vi "Q1.vi"() -> ()   [LabVIEW 2018]
uses:
  <vilib>/Analysis/geometry.llb/Point in Polygon Position.ctl
  <vilib>/Analysis/geometry.llb/Point in Polygon (Array).vi
  <vilib>/Analysis/NI_AAL_Geometry.lvlib
panel:
  out "Pendiente":dbl[](array[numeric])
  out "Puntoy":dbl[](array[numeric])
  out "Puntox":dbl[](array[numeric])
  out "Position":T1[](array[typedef]) items=["Inside", "On Boundary", "Outside"]
  out "Limite del poligono superado":bool[](array[boolean])
  out "XY Graph":cluster{"Puntox":dbl[], "Puntoy":dbl[]}[](graph)
  in  "Cluster":T2
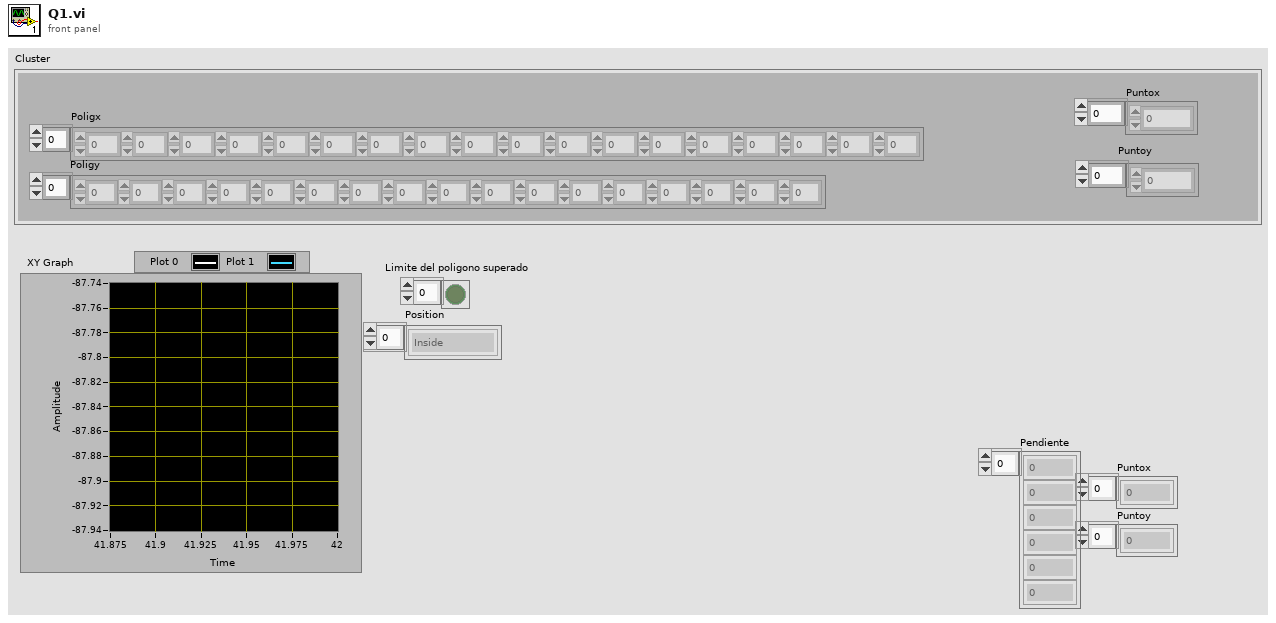
[diagram p1: front panel]
types:
  T1 = typedef "NI_AAL_Geometry.lvlib/Point in Polygon Position.ctl" = u16
  T2 = cluster{"Poligx":dbl[], "Poligy":dbl[], "Puntox":dbl[], "Puntoy":dbl[]}
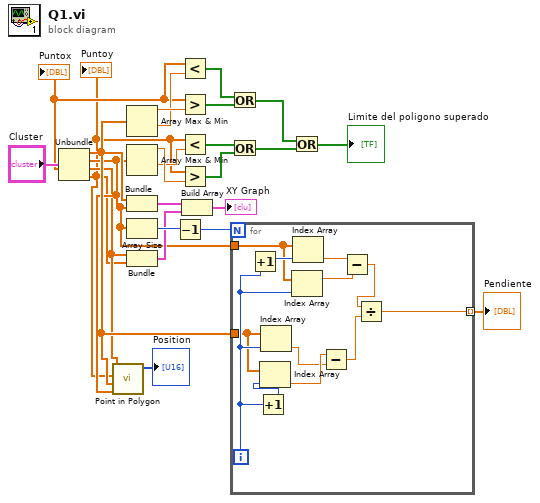
[diagram p0: block diagram]
diagram:
  n1 = Unbundle("Cluster") -> ("Poligx"=w6:dbl[], "Poligy"=w5:dbl[], "Puntox"=w4:dbl[], "Puntoy"=w3:dbl[])
  "Puntox" <- w4
  "Puntoy" <- w3
  n2 = call-poly <vilib>:"Point in Polygon.vi"("Polygon Y"=w5, "Polygon X"=w6, "Y"=w3, "X"=w4) -> ("Position"=→"Position":T1[])  [unwired: 6 in, 1 out]
  n3 = Array Max & Min(array=w6) -> (max value=w21:dbl, min value=w13:dbl)  [unwired: 2 out]
  n4 = Array Max & Min(array=w5) -> (max value=w19:dbl, min value=w14:dbl)  [unwired: 2 out]
  n5 = Bundle("Poligx"=w6, "Poligy"=w5) -> (w8:cluster{"Poligx":dbl[], "Poligy":dbl[]})  [unwired: 1 in]
  n6 = Array Size(array=w5) -> (size(s)=w10:i32)
  n7 = Bundle("Puntox"=w4, "Puntoy"=w3) -> (w7:cluster{"Puntox":dbl[], "Puntoy":dbl[]})  [unwired: 1 in]
  n8 = Decrement(x=w10) -> (x-1=w9:i32)
  n9 = Less?(x=w4, y=w13) -> (x < y?=w22:bool[])
  n10 = Greater?(x=w4, y=w21) -> (0:w20:bool[])
  n11 = Less?(x=w3, y=w14) -> (x < y?=w18:bool[])
  n12 = Greater?(x=w3, y=w19) -> (0:w17:bool[])
  n13 = Build Array(w8, w7) -> (→"XY Graph":cluster{"Puntox":dbl[], "Puntoy":dbl[]}[])
  n14 = Or(x=w22, y=w20) -> (x .or. y?=w15:bool[])
  n15 = Or(x=w18, y=w17) -> (x .or. y?=w16:bool[])
  n16 = for {
    N: w9 -> [_]
    tunnel: w5 -> [w34]
    tunnel: w6 -> [w30]
    tunnel: [w24] -> w1 mode=indexing
    i -> [w31]
    n17 = Increment(x=w31) -> (x+1=w35:i32)
    n18 = Increment(x=w31) -> (x+1=w27:i32)
    n19 = Index Array(array=w30, index=w27) -> (element=w26:dbl)
    n20 = Index Array(array=w30, index=w31) -> (element=w25:dbl)
    n21 = Index Array(array=w34, index=w31) -> (element=w32:dbl)
    n22 = Index Array(array=w34, index=w35) -> (element=w33:dbl)
    n23 = Subtract(x=w26, y=w25) -> (x-y=w28:dbl)
    n24 = Subtract(x=w33, y=w32) -> (x-y=w29:dbl)
    n25 = Divide(x=w29, y=w28) -> (x/y=w24:dbl)
  }
  "Pendiente" <- w1
  n26 = Or(x=w15, y=w16) -> (x .or. y?=→"Limite del poligono superado":bool[])
